vi "ztscopeM Channel Enable.vi"(8 "error in":errorcluster, 9 "State":i32(ring)=1 items=["Enable"=1, "Disable"=0], 10 "Channel":i32(ring) items=["Input Channel 1", "Input Channel 2", "Input Channel 3", "Input Channel 4"], 11 "Instrument Handle In":i32) -> (0 "error out":errorcluster, 3 "Instrument Handle Out":i32)   [LabVIEW 2013]
doc: "Enable or Disable the selected input channel."
uses:
  ztscopeM.dll
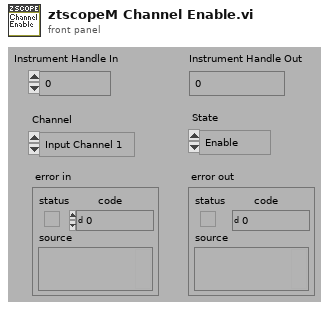
[diagram p1: front panel]
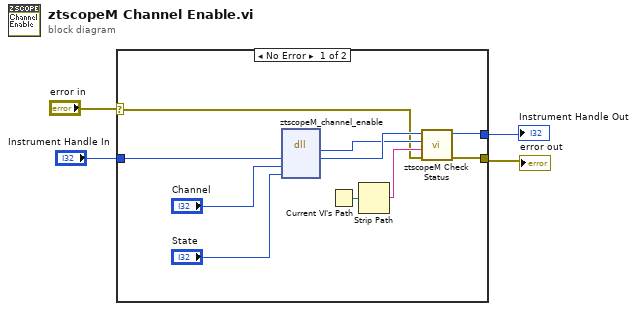
[diagram p0: block diagram]
diagram:
  n1 = case shown="No Error" "error in" {
    selector: "error in" -> [w5 w16]
    tunnel: [w9 w16] -> w1
    tunnel: "Instrument Handle In" -> [w14 w15]
    tunnel: [w8 w15] -> w3
    frame No Error {
      n2 = dll-call lib="C:/Program Files/National Instruments/instr.lib/ztscopem/ztscopeM.dll" fn="ztscopeM_channel_enable"("instrumentHandle"=w14, "channel"="Channel", "state"="State") -> (w6:i32, "instrumentHandle"=w7:i32)  [unwired: 5 in, 2 out]
      n3 = Current VI's Path() -> (path=w11:path)
      n4 = Strip Path(path=w11) -> (name=w10:string)  [unwired: 1 out]
      n5 = call "ztscopeM Check Status.vi"("error in"=w5, "name of VI"=w10, "status"=w6, "instrument handle in"=w7) -> ("error out"=w9:errorcluster, "instrument handle out"=w8:i32)  [unwired: 2 in]
    }
    frame Error {
    }
  }
  "Instrument Handle Out" <- w3
  "error out" <- w1
